vi "SVL Calibrate Accelerometer (DAQmx).vi"(0 "DAQmx physical channel":tag, 1 "calibration settings":T8={"calibration value [EU rms]"=1.0, "calibration frequency [Hz]"=159.15494309189535} {"calibration value [EU rms]" format="%.2f"; "calibration frequency [Hz]" format="%.2f"}, 2 "channel configuration":T7={"maximum value (V)"=1.0, "minimum value (V)"=-1.0, "terminal configuration"=-1} {"terminal configuration" items=["Default"=-1, "RSE"=10083, "NRSE"=10078, "Differential"=10106, "Pseudodifferential"=12529]; "minimum value (V)" format="%.2f"; "maximum value (V)" format="%.2f"}, 3 "enable IEPE excitation (T)":bool=TRUE, 4 "channel info":T9={"sensor sensitivity"=1000.0, "engineering units"=3, "dB reference"=1.0, "custom label"="EU", "weighting filter"=0, "pregain"=0.0} {"pregain" format="%.2f"; "weighting filter" items=["Linear", "A-weighting", "B-weighting", "C-weighting", "ITU-R 468-4", "Dolby", "CCITT", "C-message", "Wb", "Wc", "Wd", "We", "Wf", "Wh", "Wj", "Wk", "Wm", "AES17 20 kHz lowpass", "AES17 40 kHz lowpass", "AES17 20 kHz highpass", "AES17 40 kHz highpass"]; "dB reference" format="%^.1e"; "engineering units" items=["custom..."=0, "V"=1, "A"=21, "C"=30, "pC"=31, "s"=32, "-"=29, "Pa"=2, "N"=20, "g"=3, "m/s^2"=4, "m/s"=5, "m"=6, "mm/s"=12, "mm"=13, "micron/s"=14, "micron"=15, "in/s^2"=7, "in/s"=8, "in"=9, "mil/s"=10, "mil"=11, "rad/s^2"=16, "rad/s"=17, "rad"=18, "deg/s^2"=26, "deg/s"=27, "deg"=28, "RPM"=22, "cycle/s^2"=23, "Hz"=24, "cycle"=25, "strain"=19]; "sensor sensitivity" format="%#_5f"}, 5 "error in (no error)":errorcluster, 6 "sampling frequency [Hz]":dbl=25600.0 format="%.2f", 7 "self calibrate device (F)":bool, 8 "duration [s]":dbl=1.0 format="%.2f", 9 "time to settle [s]":dbl format="%_2f", 11 "IEPE current [mA]":dbl=2.0 format="%_2f") -> (10 "power spectrum":cluster{"x0":dbl, "dx":dbl, "magnitude":dbl[]}(graph), 12 "spectrum info":T1={"channel name"="", "description"="", "x-axis units"=0, "spectral info"={"spectrum type"=enum."Power [Magnitude^2]", "linear/dB"=enum."linear", "window"=0, "window size"=0, "FFT size"=0}, "engineering units"=1, "custom label"="", "dB reference [EU]"=0.0, "peak units"=enum."rms", "weighting filter"=0, "spectral density?"=FALSE, "unit label"="", "spectrum skewed?"=FALSE, "complimentary spectrum units"=enum."none"} {"x-axis units" items=["Time (s)"=0, "Frequency-CB (Hz)"=1, "Frequency-CPB (Hz)"=1248, "Frequency-Arbitrary (Hz)"=2357, "Quefrency (s)"=2, "Revolutions (rev)"=3, "Order"=4, "Speed (RPM)"=11, "Speed (rad/s)"=21, "Index"=65535]; "weighting filter" items=["Linear", "A-weighting", "B-weighting", "C-weighting", "ITU-R 468-4", "Dolby", "CCITT", "C-message", "Wb", "Wc", "Wd", "We", "Wf", "Wh", "Wj", "Wk", "Wm", "AES17 20 kHz lowpass", "AES17 40 kHz lowpass", "AES17 20 kHz highpass", "AES17 40 kHz highpass"]; "dB reference [EU]" format="%.2f"; "engineering units" items=["custom..."=0, "V"=1, "A"=21, "C"=30, "pC"=31, "s"=32, "-"=29, "Pa"=2, "N"=20, "g"=3, "m/s^2"=4, "m/s"=5, "m"=6, "mm/s"=12, "mm"=13, "micron/s"=14, "micron"=15, "in/s^2"=7, "in/s"=8, "in"=9, "mil/s"=10, "mil"=11, "rad/s^2"=16, "rad/s"=17, "rad"=18, "deg/s^2"=26, "deg/s"=27, "deg"=28, "RPM"=22, "cycle/s^2"=23, "Hz"=24, "cycle"=25, "strain"=19]; "spectral info"."window" items=["None "=0, "Hanning"=1, "Hamming"=2, "Blackman-Harris"=3, "Exact Blackman"=4, "Blackman"=5, "Flat Top"=6, "4 Term B-Harris "=7, "7 Term B-Harris"=8, "Low Sidelobe"=9, "Force - Exponential"=10, "Gaussian"=62]}, 14 "calibrated sensor sensitivity [mV/g]":dbl=nan format="%.2g", 15 "calibrated channel info":T9={"sensor sensitivity"=nan, "engineering units"=3, "dB reference"=1.0, "custom label"="EU", "weighting filter"=0, "pregain"=0.0} {"pregain" format="%.2f"; "weighting filter" items=["Linear", "A-weighting", "B-weighting", "C-weighting", "ITU-R 468-4", "Dolby", "CCITT", "C-message", "Wb", "Wc", "Wd", "We", "Wf", "Wh", "Wj", "Wk", "Wm", "AES17 20 kHz lowpass", "AES17 40 kHz lowpass", "AES17 20 kHz highpass", "AES17 40 kHz highpass"]; "dB reference" format="%^.1e"; "engineering units" items=["custom..."=0, "V"=1, "A"=21, "C"=30, "pC"=31, "s"=32, "-"=29, "Pa"=2, "N"=20, "g"=3, "m/s^2"=4, "m/s"=5, "m"=6, "mm/s"=12, "mm"=13, "micron/s"=14, "micron"=15, "in/s^2"=7, "in/s"=8, "in"=9, "mil/s"=10, "mil"=11, "rad/s^2"=16, "rad/s"=17, "rad"=18, "deg/s^2"=26, "deg/s"=27, "deg"=28, "RPM"=22, "cycle/s^2"=23, "Hz"=24, "cycle"=25, "strain"=19]; "sensor sensitivity" format="%#_5f"}, 16 "amplitude [V rms]":dbl=nan format="%.4f", 17 "frequency [Hz]":dbl=nan format="%.2f", 19 "error out":errorcluster)   [LabVIEW 2017, in "SoundVib_Calibration.lvlib"]
doc: "Performs an end-to-end calibration on the selected channel by measuring the actual sensitivity of the sensor connected to the channel and returns the measured sensor sensitivity."
uses:
  <vilib>/addons/Sound and Vibration/svt_Calibration/SoundVib_Calibration.lvlib
  <vilib>/addons/_NISVFA/_Shared subVIs/Controls/svc_Channel Info.ctl
  <vilib>/addons/_NISVFA/_Shared subVIs/Controls/svc_Engineering Units Text Ring.ctl
  <vilib>/addons/_NISVFA/_Shared subVIs/Controls/svc_Weighting Filter Text Ring.ctl
  <vilib>/addons/_NISVFA/_Shared subVIs/Controls/svc_Spectrum Info.ctl
  <vilib>/addons/_NISVFA/_Shared subVIs/Controls/svc_X-Axis Units.ctl
  <vilib>/addons/_NISVFA/_Shared subVIs/Controls/svc_Spectrum Type.ctl
  <vilib>/addons/_NISVFA/_Shared subVIs/Controls/svc_Complimentary Spectrum Units.ctl
  <vilib>/addons/_NISVFA/_Shared subVIs/Controls/svc_DSA Channel Settings.ctl
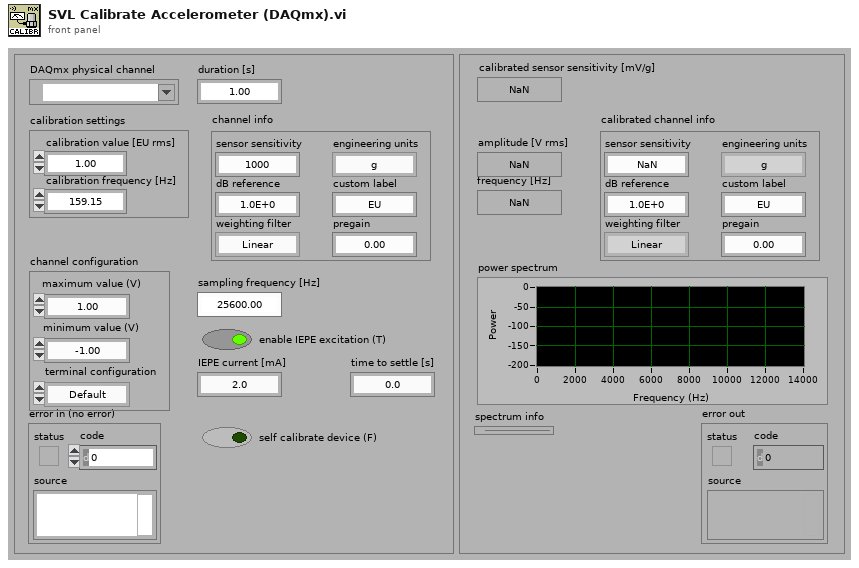
[diagram p1: front panel]
types:
  T1 = typedef "svc_Spectrum Info.ctl" = cluster{"channel name":string, "description":string, "x-axis units":T2, "spectral info":cluster{"spectrum type":T3, "linear/dB":enum16{"linear", "dB"}, "window":u16, "window size":i32, "FFT size":i32}, "engineering units":T4, "custom label":string, "dB reference [EU]":dbl, "peak units":enum16{"rms", "peak", "peak-peak"}, "weighting filter":T5, "spectral density?":bool, "unit label":string, "spectrum skewed?":bool, "complimentary spectrum units":T6}
  T2 = typedef "svc_X-Axis Units.ctl" = u16
  T3 = typedef "svc_Spectrum Type.ctl" = enum16{"FFT Spectrum [complex]", "Amplitude [Magnitude]", "Power [Magnitude^2]", "Cross Spectrum [complex]", "Frequency Response [Complex]"}
  T4 = typedef "svc_Engineering Units Text Ring.ctl" = u16
  T5 = typedef "svc_Weighting Filter Text Ring.ctl" = u16
  T6 = typedef "svc_Complimentary Spectrum Units.ctl" = enum16{"none", "radians", "degrees", "cycles", "imaginary"}
  T7 = cluster{"maximum value (V)":dbl, "minimum value (V)":dbl, "terminal configuration":i32}
  T8 = cluster{"calibration value [EU rms]":dbl, "calibration frequency [Hz]":dbl}
  T9 = typedef "svc_Channel Info.ctl" = cluster{"sensor sensitivity":dbl, "engineering units":T4, "dB reference":dbl, "custom label":string, "weighting filter":T5, "pregain":dbl}
  T10 = typedef "svc_DSA Channel Settings.ctl" = cluster{"coupling":i32, "enable IEPE excitation":bool, "IEPE current [mA]":dbl}
  T11 = cluster{"calibration value [EUrms]":dbl, "calib. value is in dB (T)":bool, "calibration frequency [Hz]":dbl, "frequency tolerance [%]":dbl}
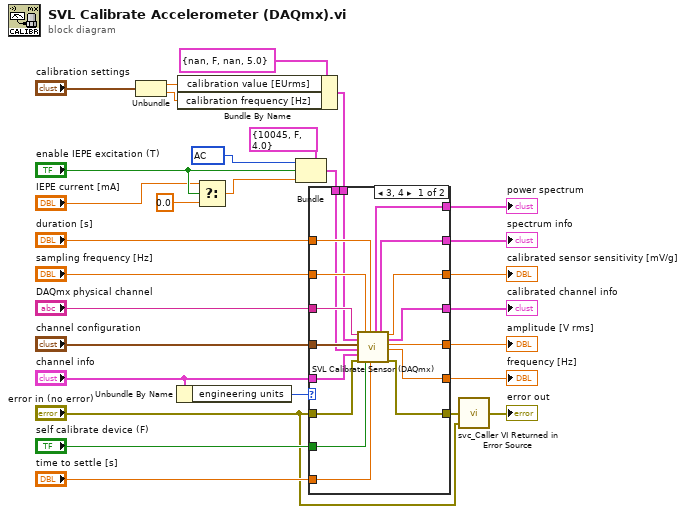
[diagram p0: block diagram]
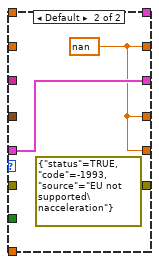
[diagram p2: hidden frame]
diagram:
  w13 = 10045 items=["AC"=10045, "DC"=10050, "GND"=10066] ("coupling")
  n1 = Unbundle("calibration settings") -> ("calibration value [EU rms]"=w19:dbl, "calibration frequency [Hz]"=w18:dbl)
  n2 = Unbundle By Name("channel info") -> ("engineering units"=w9:T4)
  n3 = Bundle By Name(cluster=T11 {"calibration value [EUrms]"=nan, "calib. value is in dB (T)"=FALSE, "calibration frequency [Hz]"=nan, "frequency tolerance [%]"=5.0} ("calibration settings"), "calibration value [EUrms]"=w19, "calibration frequency [Hz]"=w18) -> (w23:T11)
  n4 = Select(t="IEPE current [mA]", s="enable IEPE excitation (T)", f=0.0) -> (s? t:f=w5:dbl)
  n5 = Bundle(cluster=T10 {"coupling"=10045, "enable IEPE excitation"=FALSE, "IEPE current [mA]"=4.0} ("DSA channel settings"), "coupling"=w13, "enable IEPE excitation"="enable IEPE excitation (T)", "IEPE current [mA]"=w5) -> (w21:T10)
  n6 = case shown="3, 4" w9 {
    tunnel: "error in (no error)" -> [w46 _]
    tunnel: [w45 errorcluster {"status"=TRUE, "code"=-1993, "source"="EU not supported\nacceleration"} ("error out")] -> w12
    tunnel: "self calibrate device (F)" -> [w44 _]
    tunnel: "time to settle [s]" -> [w43 _]
    tunnel: "DAQmx physical channel" -> [w42 _]
    tunnel: "sampling frequency [Hz]" -> [w41 _]
    tunnel: "duration [s]" -> [w40 _]
    tunnel: w23 -> [w39 _]
    tunnel: "channel configuration" -> [w38 _]
    tunnel: w21 -> [w37 _]
    tunnel: [w36 w48] -> w17
    tunnel: [w35 w49] -> w16
    tunnel: [w34 w48] -> w15
    tunnel: [w33 w48] -> w14
    tunnel: "channel info" -> [w32 w49]
    tunnel: [w31 _] -> w4
    tunnel: [w30 _] -> w3
    frame 3, 4 {
      n7 = call <vilib>:"SVL Calibrate Sensor (DAQmx).vi"("DAQmx physical channel"=w42, "calibration settings"=w39, "channel configuration"=w38, "DSA channel settings"=w37, "channel info"=w32, "error in (no error)"=w46, "sampling frequency [Hz]"=w41, "self calibrate device (F)"=w44, "duration [s]"=w40, "time to settle [s]"=w43) -> ("power spectrum"=w31:cluster{"x0":dbl, "dx":dbl, "magnitude":dbl[]}, "spectrum info"=w30:T1, "calibrated sensor sensitivity [mV/EU]"=w36:dbl, "calibrated channel info"=w35:T9, "amplitude [V rms]"=w34:dbl, "frequency [Hz]"=w33:dbl, "error out"=w45:errorcluster)  [unwired: 3 in]
    }
    frame Default {
      w48 = nan ("calibrated sensor sensitivity [mV/EU]")
    }
  }
  "amplitude [V rms]" <- w15
  "calibrated sensor sensitivity [mV/g]" <- w17
  "frequency [Hz]" <- w14
  "calibrated channel info" <- w16
  "power spectrum" <- w4
  "spectrum info" <- w3
  n8 = call <vilib>:"svc_Caller VI Returned in Error Source.vi"("warning input to caller"="error in (no error)", "error in (no error)"=w12) -> ("error out"=→"error out":errorcluster)  [unwired: 3 in]
